vi "Plot_build_legend.vi"(7 "Y_id":i32, 8 "X_id":i32, 9 "Exp_params":T3={"filename"="201612181913", "ExpFilePath"=path "C:/Documents and Settings/Bauerle/Mes documents/takada/HBT6/201612181913.h5", "File Ref list"=[16777217, 33554433, 16777216, 33554432], "sweep_dim"=[11, 61, 61], "sweep_list"=["suq", "ruq", "rlq", "slq", "sur", "rur", "rlr", "slr", "suc", "ruc", "rlc", "slc"], "readout_list"=["sud", "rud", "rld", "sld"], "Sweep instrument bools"=[[0, 0], [0, 0], [0, 0], [0, 0], [0, 0], [0, 0], [0, 0], [0, 0], [0, 0], [0, 0], [0, 0], [0, 0], [0, 0], [0, 0], [0, 0], [0, 0], [0, 0], [0, 0], [0, 0], [0, 0], [0, 0], [0, 0], [0, 0], [0, 0], [0, 0], [0, 0], [0, 0], [0, 0], [0, 0], [0, 0], [0, 0], [0, 0], [0, 0], [0, 0], [0, 0], [0, 0], [0, 0], [0, 0], [0, 0], [0, 0], [0, 0]], "Read out instrument bools"=[[1, 0]], "Experimental bool list"=[TRUE, TRUE], "Initial move"=[{"Name"="None", "kind"=100, "Value"=0.0}], "FPGA Ref"=refnum, "Inst_parameters"={"ConfigFilePath"=path "\\\\10.0.0.7\\takada2/DATA/HBT6/data/Configs/conf_20161218_fc_load.h5", "Inst_list"=["ADC", "AWG", "Freq", "Power", "sus", "rus", "rls", "sls", "suq", "suu", "sur", "suc", "sul", "ruq", "ruu", "rur", "ruc", "rul", "rlq", "rlu", "rlr", "rlc", "rll", "slq", "slu", "slr", "slc", "sll", "tu", "t", "tl", "fast_sequence", "4:7", "suc_load", "sur_load", "ruc_load", "rur_load", "rlc_load", "rlr_load", "slc_load", "slr_load", "load_time"], "fast_mode"=[1, 0], "Wait_times"=[1, 1, 1, 1], "Inst_array"=[{"Kind"=0, "Strings"=["ADC", "", "V", "sud;rud;rld;sld", "nA;nA;nA;nA", "100.0;100.0;100.0;100.0"], "uint64s"=[5, 4, 250000, 1, 100, 10106, 1000000, 1, 0, 1], "Doubles"=[1.0], "DAQmx take out list"=[]}, {"Kind"=7, "Strings"=["AWG", "10.0.0.4", "", "C:\\Documents and Settings\\Bauerle\\Mes documents\\Bautze\\FPGA-clean_works_1.13.6_batchtest\\Python\\AWG", "dummy", "SAWnstrig_v4.py"], "uint64s"=[2, 0, 0, 3, 0, 0, 0, 0, 0, 0, 0, 0, 0, 0], "Doubles"=[1200000000.0, 1.0, 0.0, 1.0, 0.0, 1.0, 0.0, 1.0, 0.0, 1.0, 0.0, 1.0, 0.0], "DAQmx take out list"=[]}, {"Kind"=6, "Strings"=["Freq", "0:19", "GHz"], "uint64s"=[1, 0, 0, 0, 2, 0, 0, 0], "Doubles"=[2.0, -30.0, 200.0, 100.0, 0.0, 6.000999927520752, 9.000000318337698e-06, 30.0, -145.0], "DAQmx take out list"=[]}, {"Kind"=6, "Strings"=["Power", "0:19", "GHz"], "uint64s"=[1, 0, 1, 0, 2, 0, 0, 1], "Doubles"=[2.0, -30.0, 200.0, 100.0, 0.0, 6.000999927520752, 9.000000318337698e-06, 30.0, -145.0], "DAQmx take out list"=[]}, {"Kind"=4, "Strings"=["sus", "10.0.0.2", "mV"], "uint64s"=[0, 1], "Doubles"=[1.0, -1.0, 1.0, -1.0, 1.0], "DAQmx take out list"=[]}, {"Kind"=4, "Strings"=["rus", "10.0.0.2", "mV"], "uint64s"=[0, 2], "Doubles"=[1.0, -1.0, 1.0, -1.0, 1.0], "DAQmx take out list"=[]}, {"Kind"=4, "Strings"=["rls", "10.0.0.2", "mV"], "uint64s"=[0, 3], "Doubles"=[1.0, -1.0, 1.0, -1.0, 1.0], "DAQmx take out list"=[]}, {"Kind"=4, "Strings"=["sls", "10.0.0.2", "mV"], "uint64s"=[0, 4], "Doubles"=[1.0, -1.0, 1.0, -1.0, 1.0], "DAQmx take out list"=[]}, {"Kind"=4, "Strings"=["suq", "10.0.0.2", "V"], "uint64s"=[0, 5], "Doubles"=[0.30000001192092896, -2.0, 1.0, -1.0, 1.0], "DAQmx take out list"=[]}, {"Kind"=4, "Strings"=["suu", "10.0.0.2", "V"], "uint64s"=[0, 6], "Doubles"=[0.30000001192092896, -2.0, 1.0, -1.0, 1.0], "DAQmx take out list"=[]}, {"Kind"=4, "Strings"=["sur", "10.0.0.2", "V"], "uint64s"=[0, 7], "Doubles"=[0.30000001192092896, -2.0, 1.0, -1.0, 1.0], "DAQmx take out list"=[]}, {"Kind"=4, "Strings"=["suc", "10.0.0.2", "V"], "uint64s"=[1, 0], "Doubles"=[0.30000001192092896, -2.0, 1.0, -1.0, 1.0], "DAQmx take out list"=[]}, {"Kind"=4, "Strings"=["sul", "10.0.0.2", "V"], "uint64s"=[1, 1], "Doubles"=[0.30000001192092896, -2.0, 1.0, -1.0, 1.0], "DAQmx take out list"=[]}, {"Kind"=4, "Strings"=["ruq", "10.0.0.2", "V"], "uint64s"=[1, 2], "Doubles"=[0.30000001192092896, -2.0, 1.0, -1.0, 1.0], "DAQmx take out list"=[]}, {"Kind"=4, "Strings"=["ruu", "10.0.0.2", "V"], "uint64s"=[1, 3], "Doubles"=[0.30000001192092896, -2.0, 1.0, -1.0, 1.0], "DAQmx take out list"=[]}, {"Kind"=4, "Strings"=["rur", "10.0.0.2", "V"], "uint64s"=[1, 5], "Doubles"=[0.30000001192092896, -2.0, 1.0, -1.0, 1.0], "DAQmx take out list"=[]}, {"Kind"=4, "Strings"=["ruc", "10.0.0.2", "V"], "uint64s"=[1, 6], "Doubles"=[0.30000001192092896, -2.0, 1.0, -1.0, 1.0], "DAQmx take out list"=[]}, {"Kind"=4, "Strings"=["rul", "10.0.0.2", "V"], "uint64s"=[1, 7], "Doubles"=[0.30000001192092896, -2.0, 1.0, -1.0, 1.0], "DAQmx take out list"=[]}, {"Kind"=4, "Strings"=["rlq", "10.0.0.2", "V"], "uint64s"=[2, 0], "Doubles"=[0.30000001192092896, -2.0, 1.0, -1.0, 1.0], "DAQmx take out list"=[]}, {"Kind"=4, "Strings"=["rlu", "10.0.0.2", "V"], "uint64s"=[2, 1], "Doubles"=[0.30000001192092896, -2.0, 1.0, -1.0, 1.0], "DAQmx take out list"=[]}, {"Kind"=4, "Strings"=["rlr", "10.0.0.2", "V"], "uint64s"=[2, 2], "Doubles"=[0.30000001192092896, -2.0, 1.0, -1.0, 1.0], "DAQmx take out list"=[]}, {"Kind"=4, "Strings"=["rlc", "10.0.0.2", "V"], "uint64s"=[2, 3], "Doubles"=[0.30000001192092896, -2.0, 1.0, -1.0, 1.0], "DAQmx take out list"=[]}, {"Kind"=4, "Strings"=["rll", "10.0.0.2", "V"], "uint64s"=[2, 4], "Doubles"=[0.30000001192092896, -2.0, 1.0, -1.0, 1.0], "DAQmx take out list"=[]}, {"Kind"=4, "Strings"=["slq", "10.0.0.2", "V"], "uint64s"=[2, 5], "Doubles"=[0.30000001192092896, -2.0, 1.0, -1.0, 1.0], "DAQmx take out list"=[]}, {"Kind"=4, "Strings"=["slu", "10.0.0.2", "V"], "uint64s"=[2, 6], "Doubles"=[0.30000001192092896, -2.0, 1.0, -1.0, 1.0], "DAQmx take out list"=[]}, {"Kind"=4, "Strings"=["slr", "10.0.0.2", "V"], "uint64s"=[2, 7], "Doubles"=[0.30000001192092896, -2.0, 1.0, -1.0, 1.0], "DAQmx take out list"=[]}, {"Kind"=4, "Strings"=["slc", "10.0.0.2", "V"], "uint64s"=[3, 0], "Doubles"=[0.30000001192092896, -2.0, 1.0, -1.0, 1.0], "DAQmx take out list"=[]}, {"Kind"=4, "Strings"=["sll", "10.0.0.2", "V"], "uint64s"=[3, 1], "Doubles"=[0.30000001192092896, -2.0, 1.0, -1.0, 1.0], "DAQmx take out list"=[]}, {"Kind"=4, "Strings"=["tu", "10.0.0.2", "V"], "uint64s"=[3, 2], "Doubles"=[0.30000001192092896, -2.0, 1.0, -1.0, 1.0], "DAQmx take out list"=[]}, {"Kind"=4, "Strings"=["t", "10.0.0.2", "V"], "uint64s"=[3, 3], "Doubles"=[0.30000001192092896, -2.0, 1.0, -1.0, 1.0], "DAQmx take out list"=[]}, {"Kind"=4, "Strings"=["tl", "10.0.0.2", "V"], "uint64s"=[3, 4], "Doubles"=[0.30000001192092896, -2.0, 1.0, -1.0, 1.0], "DAQmx take out list"=[]}, {"Kind"=9, "Strings"=["fast_sequence", "10.0.0.2", "V"], "uint64s"=[6661, 300, 100, 0, 7, 8, 5, 13, 14, 10, 18, 19, 16, 23, 24, 21, 26, 27, 28, 39, 0], "Doubles"=[1.0, -1.0, -1.0, -1.0], "DAQmx take out list"=[]}, {"Kind"=4, "Strings"=["4:7", "10.0.0.2", "V"], "uint64s"=[4, 7], "Doubles"=[0.30000001192092896, -2.0, 1.0, -1.0, 1.0], "DAQmx take out list"=[]}, {"Kind"=10, "Strings"=["suc_load", "10.0.0.2", "V"], "uint64s"=[4, 0], "Doubles"=[0.5, -0.5], "DAQmx take out list"=[]}, {"Kind"=10, "Strings"=["sur_load", "10.0.0.2", "V"], "uint64s"=[5, 0], "Doubles"=[0.5, -0.5], "DAQmx take out list"=[]}, {"Kind"=10, "Strings"=["ruc_load", "10.0.0.2", "V"], "uint64s"=[6, 0], "Doubles"=[0.5, -0.5], "DAQmx take out list"=[]}, {"Kind"=10, "Strings"=["rur_load", "10.0.0.2", "V"], "uint64s"=[7, 0], "Doubles"=[0.5, -0.5], "DAQmx take out list"=[]}, {"Kind"=10, "Strings"=["rlc_load", "10.0.0.2", "V"], "uint64s"=[8, 0], "Doubles"=[0.5, -0.5], "DAQmx take out list"=[]}, {"Kind"=10, "Strings"=["rlr_load", "10.0.0.2", "V"], "uint64s"=[9, 0], "Doubles"=[0.5, -0.5], "DAQmx take out list"=[]}, {"Kind"=10, "Strings"=["slc_load", "10.0.0.2", "V"], "uint64s"=[10, 0], "Doubles"=[0.5, -0.5], "DAQmx take out list"=[]}, {"Kind"=10, "Strings"=["slr_load", "10.0.0.2", "V"], "uint64s"=[11, 0], "Doubles"=[0.5, -0.5], "DAQmx take out list"=[]}, {"Kind"=10, "Strings"=["load_time", "10.0.0.2", "ms"], "uint64s"=[12, 0], "Doubles"=[1000.0, -0.009999999776482582], "DAQmx take out list"=[]}]}} {"File Ref list" format="%.0x"}) -> (0 "Yunit":string, 1 "Yname":string, 2 "Xunit":string, 3 "Xname":string)   [LabVIEW 2013]
uses:
  <vilib>/addons/h5labview2/base/hid_t.ctl
  fpga-bitfile-ref.ctl
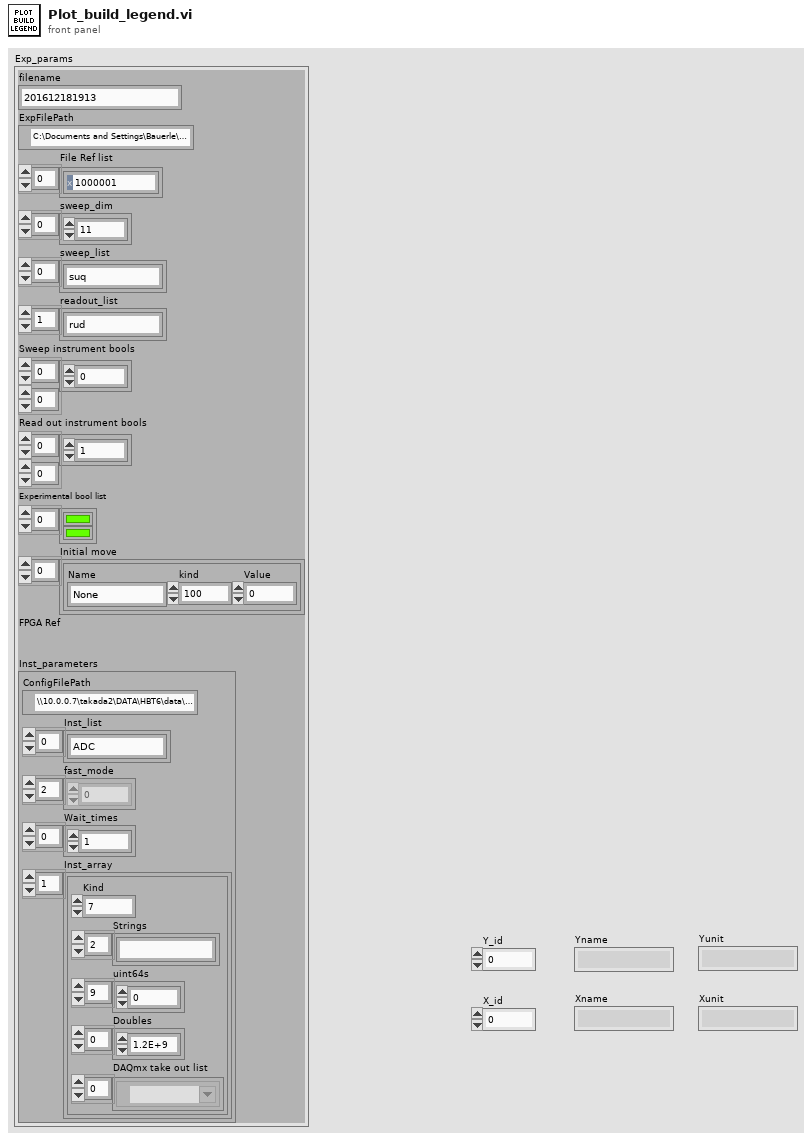
[diagram p1: front panel]
types:
  T1 = typedef "hid_t.ctl" = i32
  T2 = typedef "fpga-bitfile-ref.ctl" = refnum<k20>
  T3 = cluster{"filename":string, "ExpFilePath":path, "File Ref list":T1[], "sweep_dim":u64[], "sweep_list":string[], "readout_list":string[], "Sweep instrument bools":u64[][], "Read out instrument bools":u64[][], "Experimental bool list":bool[], "Initial move":cluster{"Name":string, "kind":u64, "Value":dbl}[], "FPGA Ref":T2, "Inst_parameters":cluster{"ConfigFilePath":path, "Inst_list":string[], "fast_mode":u8[], "Wait_times":u64[], "Inst_array":cluster{"Kind":u16, "Strings":string[], "uint64s":u64[], "Doubles":dbl[], "DAQmx take out list":refnum<k21>[]}[]}}
  T4 = cluster{"Kind":u16, "Strings":string[], "uint64s":u64[], "Doubles":dbl[], "DAQmx take out list":refnum<k21>[]}[]
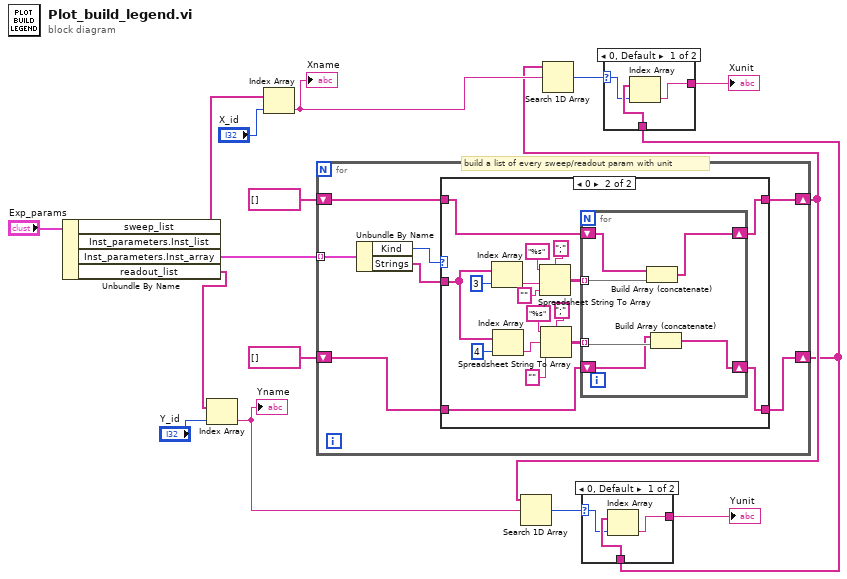
[diagram p0: block diagram]
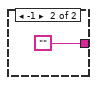
[diagram p2: hidden frame]
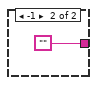
[diagram p3: hidden frame]
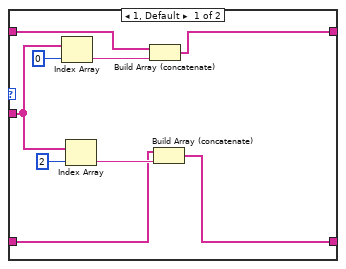
[diagram p4: hidden frame]
diagram:
  # "build a list of every sweep/readout param with unit"
  n1 = Unbundle By Name("Exp_params") -> ("sweep_list"=w13:string[], "Inst_parameters.Inst_array"=w10:T4, "readout_list"=w1:string[])  [unwired: 1 out]
  n2 = Index Array(array=w1, index="Y_id") -> (element=w5:string)
  "Yname" <- w5
  n3 = Index Array(array=w13, index="X_id") -> (element=w9:string)
  "Xname" <- w9
  n4 = for {
    shift-right: [w20] -> w4
    shift-left: string[] [] -> [w21]
    shift-right: [w18] -> w3
    shift-left: string[] [] -> [w19]
    tunnel: w10 -> [w23] mode=indexing
    n5 = Unbundle By Name(w23) -> ("Kind"=w17:u16, "Strings"=w22:string[])
    n6 = case shown="0" w17 {
      tunnel: w22 -> [w26 w47]
      tunnel: w21 -> [w31 w38]
      tunnel: [w29 w34] -> w20
      tunnel: w19 -> [w25 w35]
      tunnel: [w24 w33] -> w18
      frame 1, Default {
        n7 = Index Array(array=w26, index=0) -> (element=w30:string)
        n8 = Index Array(array=w26, index=2) -> (element=w27:string)
        n9 = Build Array (concatenate)(w31, w30) -> (w29:string[])
        n10 = Build Array (concatenate)(w25, w27) -> (w24:string[])
      }
      frame 0 {
        n11 = Index Array(array=w47, index=3) -> (element=w45:string)
        n12 = Index Array(array=w47, index=4) -> (element=w40:string)
        n13 = Spreadsheet String To Array(delimiter (Tab)=";", format string="%s", spreadsheet string=w45, array type (2D Dbl)="") -> (array=w43:string[][])
        n14 = Spreadsheet String To Array(delimiter (Tab)=";", format string="%s", spreadsheet string=w40, array type (2D Dbl)="") -> (array=w39:string[][])
        n15 = for {
          tunnel: w43 -> [w54] mode=indexing
          tunnel: w39 -> [w52] mode=indexing
          shift-right: [w53] -> w34
          shift-left: w38 -> [w55]
          shift-right: [w50] -> w33
          shift-left: w35 -> [w51]
          n16 = Build Array (concatenate)(w55, w54) -> (w53:string[])
          n17 = Build Array (concatenate)(w51, w52) -> (w50:string[])
        }
      }
    }
  }
  n18 = Search 1D Array(1D array=w4, element=w5) -> (index of element=w6:i32)  [unwired: 1 in]
  n19 = Search 1D Array(1D array=w4, element=w9) -> (index of element=w8:i32)  [unwired: 1 in]
  n20 = case shown="0, Default" w6 {
    selector: w6 -> [w57 _]
    tunnel: [w56 ""] -> w2
    tunnel: w3 -> [w58 _]
    frame 0, Default {
      n21 = Index Array(array=w58, index=w57) -> (element=w56:string)
    }
    frame -1 {
    }
  }
  "Yunit" <- w2
  n22 = case shown="0, Default" w8 {
    selector: w8 -> [w61 _]
    tunnel: [w60 ""] -> w7
    tunnel: w3 -> [w62 _]
    frame 0, Default {
      n23 = Index Array(array=w62, index=w61) -> (element=w60:string)
    }
    frame -1 {
    }
  }
  "Xunit" <- w7
